vi "main.vi"() -> ()   [LabVIEW 2014]
panel:
  in  "Registerkarte":enum32{"Seite 1"}(tab)
  in  "Boolesch":bool
  in  "Boolesch 2":bool
  in  "Boolesch 3":bool
  in  "Boolesch 4":bool
  out "Boolesch 17":bool
  in  "Stopp":bool
  out "Boolesch 18":bool
  out "Boolesch 5":bool
  out "Boolesch 6":bool
  out "Boolesch 7":bool
  out "Boolesch 8":bool
  out "Boolesch 9":bool
  out "Boolesch 10":bool
  out "Boolesch 11":bool
  out "Boolesch 12":bool
  out "Boolesch 13":bool
  out "Boolesch 14":bool
  out "Boolesch 15":bool
  out "Boolesch 16":bool
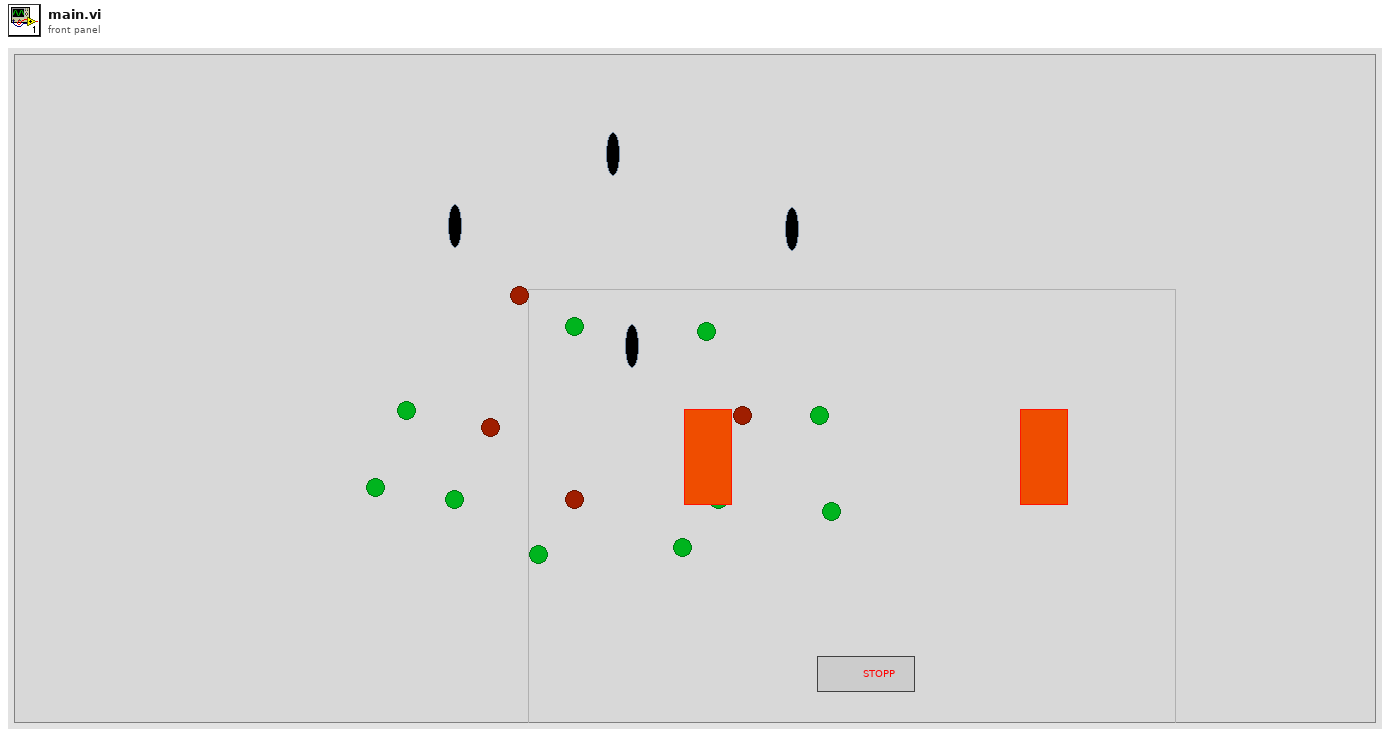
[diagram p1: front panel]
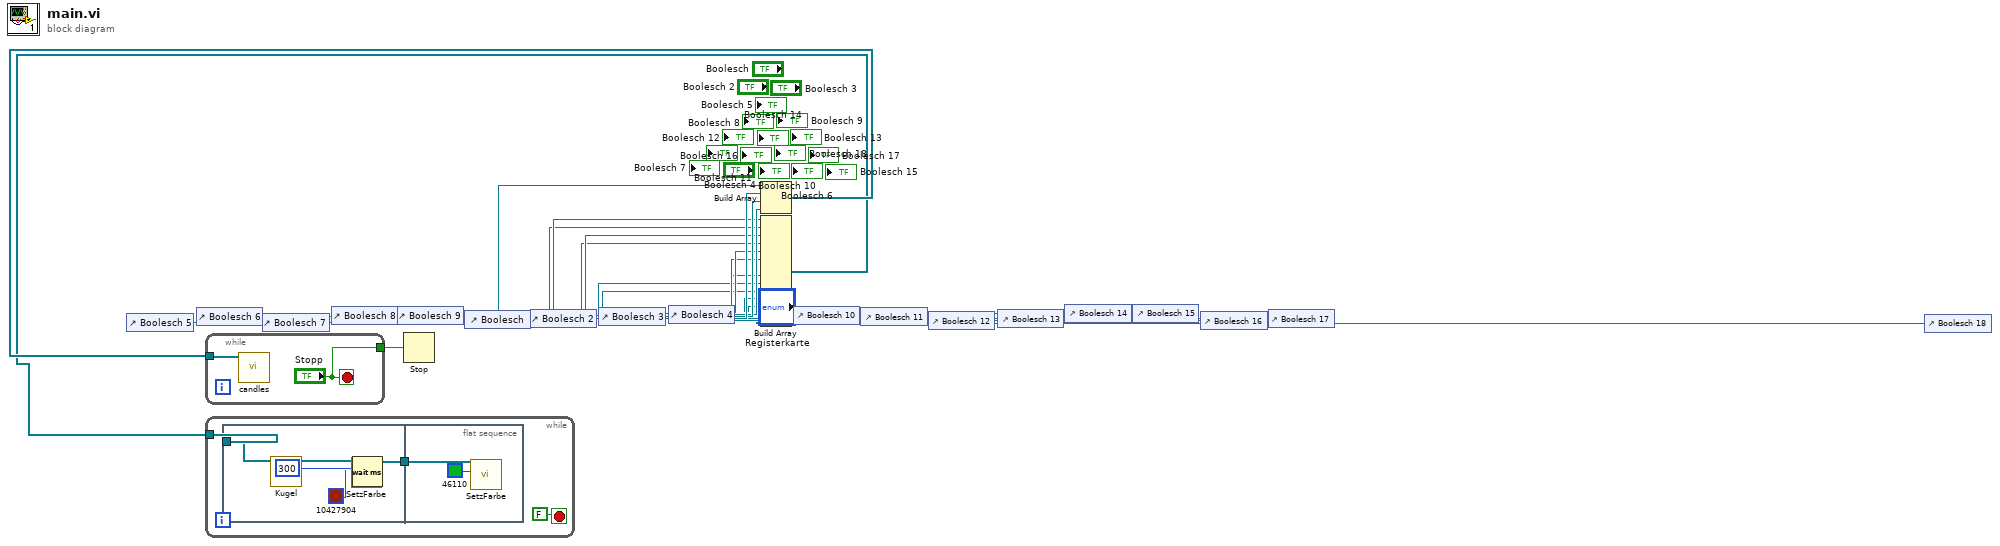
[diagram p0: block diagram]
diagram:
  n1 = control-ref of="Boolesch 5"() -> (w17:refnum<vi>)
  n2 = control-ref of="Boolesch 6"() -> (w16:refnum<vi>)
  n3 = control-ref of="Boolesch 7"() -> (w15:refnum<vi>)
  n4 = control-ref of="Boolesch 8"() -> (w14:refnum<vi>)
  n5 = control-ref of="Boolesch 9"() -> (w13:refnum<vi>)
  n6 = control-ref of="Boolesch"() -> (w21:refnum<vi>)
  n7 = control-ref of="Boolesch 2"() -> (w20:refnum<vi>)
  n8 = control-ref of="Boolesch 3"() -> (w19:refnum<vi>)
  n9 = control-ref of="Boolesch 4"() -> (w18:refnum<vi>)
  n10 = Build Array(w21, w20, w19, w18) -> (w3:refnum<vi>[])
  n11 = while {
    tunnel: w3 -> [w23]
    tunnel: ["Stopp"] -> w1
    stop <- "Stopp" stop-if-true
    n12 = call "candles.vi"("Array"=w23) -> ()  [unwired: 11 in]
  }
  n13 = Stop(stop? (T)=w1) -> ()
  n14 = control-ref of="Boolesch 10"() -> (w12:refnum<vi>)
  n15 = control-ref of="Boolesch 11"() -> (w11:refnum<vi>)
  n16 = control-ref of="Boolesch 12"() -> (w10:refnum<vi>)
  n17 = control-ref of="Boolesch 13"() -> (w9:refnum<vi>)
  n18 = control-ref of="Boolesch 14"() -> (w8:refnum<vi>)
  n19 = control-ref of="Boolesch 15"() -> (w7:refnum<vi>)
  n20 = control-ref of="Boolesch 16"() -> (w6:refnum<vi>)
  n21 = control-ref of="Boolesch 17"() -> (w5:refnum<vi>)
  n22 = control-ref of="Boolesch 18"() -> (w4:refnum<vi>)
  n23 = Build Array(w17, w16, w15, w14, w13, w12, w11, w10, w9, w8, w7, w6, w5, w4) -> (w2:refnum<vi>[])
  n24 = while {
    tunnel: w2 -> [w25]
    stop <- FALSE stop-if-true
    n25 = flat-sequence {
      tunnel: w25 -> [w27]
      tunnel: [w28] -> w26
      tunnel: w26 -> [w32]
      frame #0 {
        n26 = call "Kugel.vi"("Array (Eingang)"=w27) -> ("Array (Ausgang)"=w29:refnum<vi>[])  [unwired: 10 in]
        n27 = call "SetzFarbe.vi"("Farbfeld"=u32 10427904, "Array"=w29) -> ("Array 2"=w28:refnum<vi>[])  [unwired: 9 in]
        n28 = Wait (ms)(milliseconds to wait=u32 300 ("ms")) -> ()  [unwired: 1 out]
      }
      frame #1 {
        n29 = call "SetzFarbe.vi"("Farbfeld"=u32 46110, "Array"=w32) -> ()  [unwired: 9 in, 1 out]
      }
    }
  }
